vi "GetCurrentGrating.vi"() -> (0 "Current Grating":T1)   [LabVIEW 2015]
uses:
  GSP_GT_Global.vi
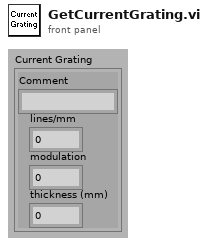
[diagram p1: front panel]
types:
  T1 = cluster{"Comment":string, "lines/mm":i32, "modulation":dbl, "thickness (mm)":dbl}
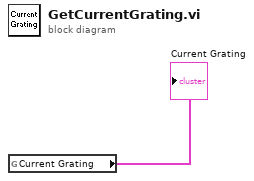
[diagram p0: block diagram]
diagram:
  n1 = global read "GSP_GT_Global.vi" "Current Grating"() -> (→"Current Grating":T1)
